vi "data.vi"() -> ()   [LabVIEW 2015]
panel:
  in  "data":u32
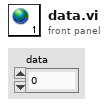
[diagram p1: front panel]
diagram:
